vi "Keithley 2002 Freq Config.vi"(1 "threshold voltage level":dbl min=-600.0 max=600.0 step=1.0 format="%^.2e", 2 "threshold voltage range (10V:1)":u16(ring)=1 items=["1 V", "10 V", "100 V", "1000 V", "TTL"], 3 "threshold current level":dbl min=-0.6 max=0.6 format="%^.2e", 4 "reference value (Hz)":dbl min=0.0 max=15000000.0 format="%^.2e", 5 "threshold current range (1mA:0)":u16(ring) items=["1 mA", "10 mA", "100 mA", "1 A"], 6 "reference (off:0)":u16(ring) items=["off", "set reference value"], 7 "resolution (5 digits:1)":u16(ring)=1 items=["4 digits", "5 digits"], 8 "error in":T1, 9 "coupling":bool=TRUE, 10 "source":bool, 11 "GPIB address":string="16") -> (0 "error out":T1)   [LabVIEW 2020]
doc: "This Vi is used to configure the settings for the Frequency measurements. The instrument can be in any mode when this mode is selected. The settings will go into effect and the instrument will go into the Frequency mode."
panel:
  # "current\nvoltage"
  # "ac\ndc"
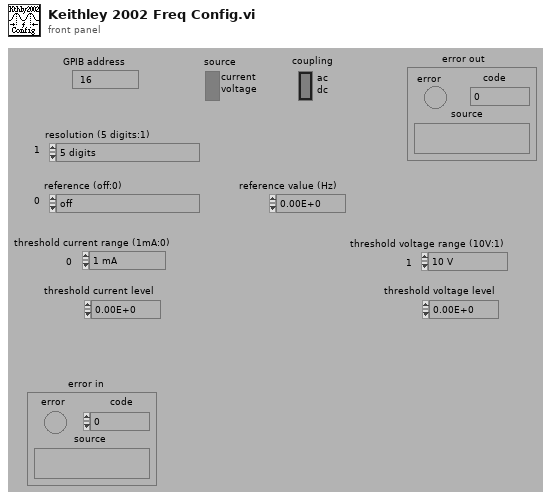
[diagram p1: front panel]
types:
  T1 = cluster{"error":bool, "code":i32, "source":string}
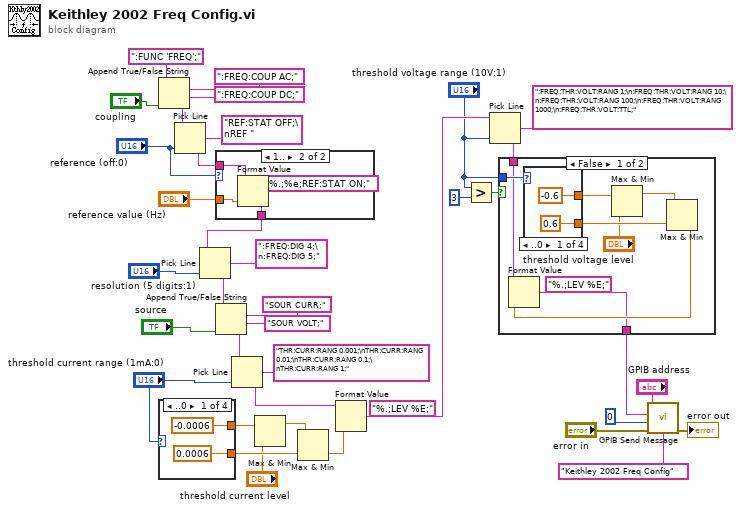
[diagram p0: block diagram]
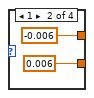
[diagram p2: hidden frame]
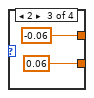
[diagram p3: hidden frame]
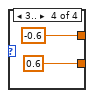
[diagram p4: hidden frame]
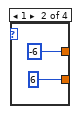
[diagram p5: hidden frame]
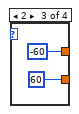
[diagram p6: hidden frame]
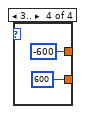
[diagram p7: hidden frame]
diagram:
  n1 = Append True/False String(1:"coupling", 2:":FREQ:COUP DC;", 3:":FREQ:COUP AC;", 4:":FUNC 'FREQ';") -> (0:w24:string)
  n2 = case shown="..0" "threshold current range (1mA:0)" {
    tunnel: [-0.0006 -0.006 -0.06 -0.6] -> w9
    tunnel: [0.0006 0.006 0.06 0.6] -> w8
    frame ..0 {
    }
    frame 1 {
    }
    frame 2 {
    }
    frame 3.. {
    }
  }
  n3 = Pick Line(string ("")=w24, multi-line string="REF:STAT OFF;\nREF ", line index="reference (off:0)") -> (output string=w36:string)
  n4 = case shown="1.." "reference (off:0)" {
    tunnel: "reference value (Hz)" -> [_ w51]
    tunnel: w36 -> [w47 w50]
    tunnel: [w47 w48] -> w23
    frame ..0 {
    }
    frame 1.. {
      n5 = Format Value(string ("")=w50, format string="%.;%e;REF:STAT ON;", value (0)=w51) -> (output string=w48:string)
    }
  }
  n6 = Pick Line(string ("")=w23, multi-line string=":FREQ:DIG 4;\n:FREQ:DIG 5;", line index="resolution (5 digits:1)") -> (output string=w19:string)
  n7 = Append True/False String(1:"source", 2:"SOUR VOLT;", 3:"SOUR CURR;", 4:w19) -> (0:w17:string)
  n8 = Pick Line(string ("")=w17, multi-line string="THR:CURR:RANG 0.001;\nTHR:CURR:RANG 0.01;\nTHR:CURR:RANG 0.1;\nTHR:CURR:RANG 1;", line index="threshold current range (1mA:0)") -> (output string=w4:string)
  n9 = Max & Min(x=w9, y="threshold current level") -> (max(x,y)=w6:dbl)  [unwired: 1 out]
  n10 = Max & Min(x=w6, y=w8) -> (min(x,y)=w5:dbl)  [unwired: 1 out]
  n11 = Format Value(string ("")=w4, format string="%.;LEV %E;", value (0)=w5) -> (output string=w14:string)
  n12 = Greater?(x="threshold voltage range (10V:1)", y=3) -> (0:w12:bool)
  n13 = Pick Line(string ("")=w14, multi-line string=":FREQ:THR:VOLT:RANG 1;\n:FREQ:THR:VOLT:RANG 10;\n:FREQ:THR:VOLT:RANG 100;\n:FREQ:THR:VOLT:RANG 1000;\n:FREQ:THR:VOLT:TTL;", line index="threshold voltage range (10V:1)") -> (output string=w10:string)
  n14 = case shown="False" w12 {
    tunnel: w10 -> [w54 w69]
    tunnel: [w52 w69] -> w2
    tunnel: "threshold voltage range (10V:1)" -> [w56 _]
    frame False {
      n15 = case shown="..0" w56 {
        tunnel: [-0.6 -6 -60 -600] -> w59
        tunnel: [0.6 6 60 600] -> w58
        frame ..0 {
        }
        frame 1 {
        }
        frame 2 {
        }
        frame 3.. {
        }
      }
      n16 = Max & Min(x=w59, y="threshold voltage level") -> (max(x,y)=w57:dbl)  [unwired: 1 out]
      n17 = Max & Min(x=w57, y=w58) -> (min(x,y)=w53:dbl)  [unwired: 1 out]
      n18 = Format Value(string ("")=w54, format string="%.;LEV %E;", value (0)=w53) -> (output string=w52:string)
    }
    frame True {
    }
  }
  n19 = call "GPIB Send Message.vi"("address string"="GPIB address", "write buffer"=w2, "source"="Keithley 2002 Freq Config", "write mode (set END:0)"=0, "error in"="error in") -> ("error out"=→"error out":T1)  [unwired: 2 in, 2 out]
